vi "MAIN.vi"(6 "ECU TYPE":u16(ring) items=["LSMD", "LSMP", "LSMRL", "LSMRR"]) -> (0 "Data By ID OK":bool, 1 "Hall Test 3 OK":bool, 2 "Sleep Request OK":bool, 3 "Hall Test 1 OK":bool, 4 "SBC OK":bool, 5 "Hall Test 2 OK":bool, 7 "Hard Reset OK":bool, 8 "BIST OK":bool, 9 "SW Version OK":bool, 10 "ECU ID OK":bool, 11 "Session OK":bool)   [LabVIEW 2023]
uses:
  Sub VIs/Global .vi
panel:
  out "Numeric Request":i32=416962034 format="%x"
  out "ReplyTracMex":string
  out "Trazabilidad":bool
  in  "Trazabilidad\nOFF  /  ON":bool
  in  "Stop":bool
  in  "Start":bool
  out "Puerto DAQ":i32
  out "Respuesta Trazabilidad":string
  out "Finish Time":string
  out "Start Time":string
  out "Status":i8
  in  "Número Serial":string
  out "Enter Brose Ext OK":bool
  out "Hall Test 3 Response":string
  out "Enter Brose Ext":string
  out "ECU Hard Reset":string
  out "Program SBC":string
  out "ID Response":string
  out "ID Request":string
  out "Tester Present OK":bool
  out "Hall Test 2 Response":string
  out "Hall Test 1 Response":string
  out "Supply Voltage ADC Response":string
  out "Self Test BIST":string
  out "Sleep Request Response":string
  out "Read Data By ID":string
  out "Verify ECU ID String":string
  out "Verify SW Version":string
  out "Tester Present Command":string
  out "Enter Brose EOL Ext Session":string
  # "*Revisar debido a cambio en respuesta"
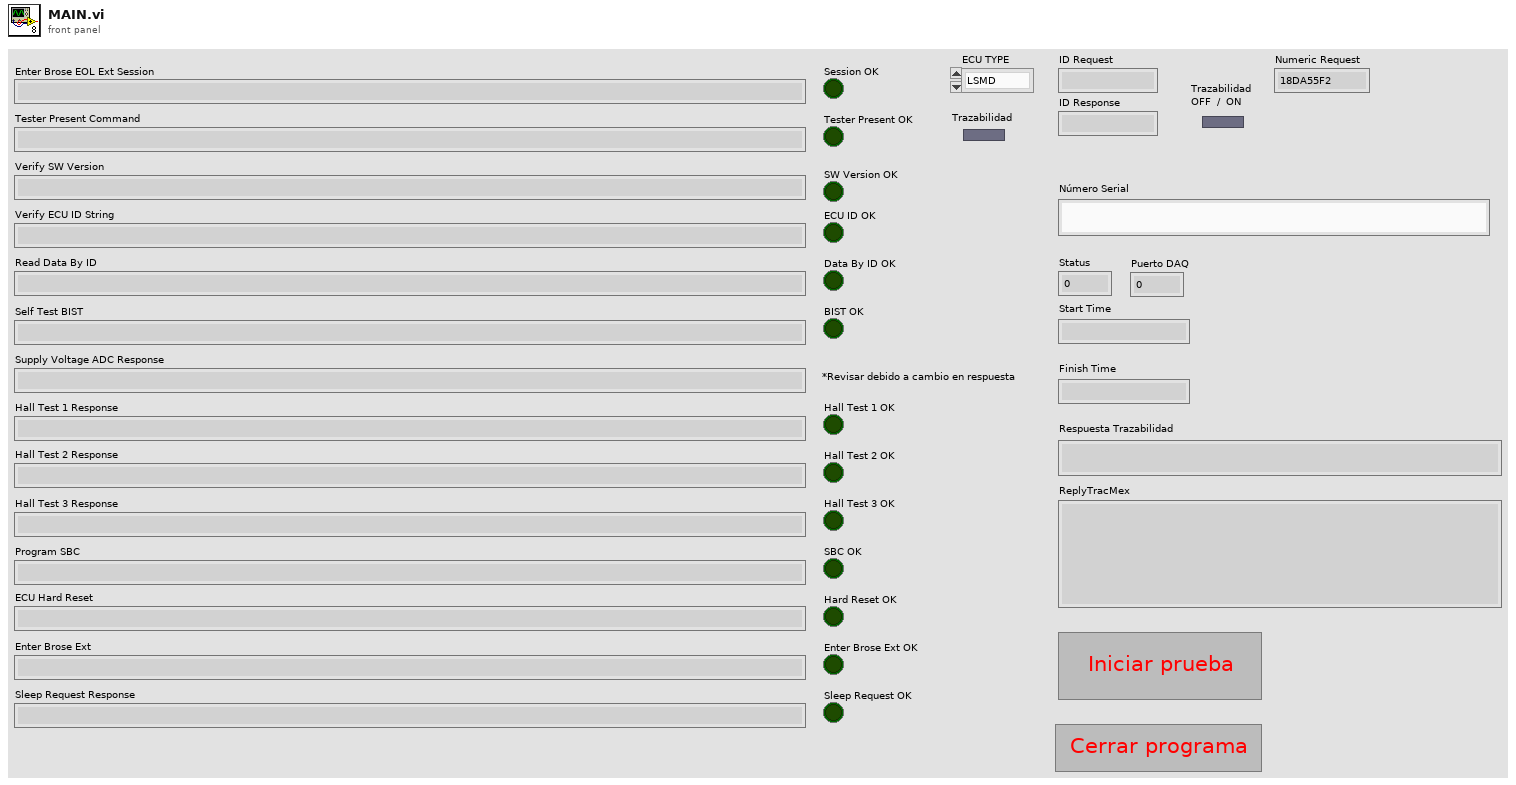
[diagram p1: front panel]
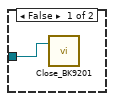
[diagram p2: hidden frame]
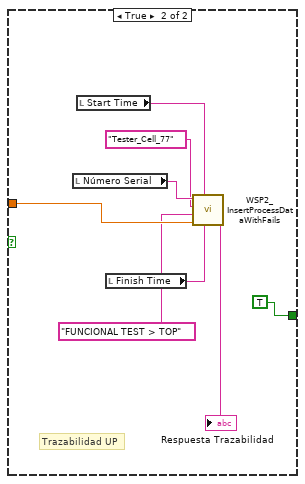
[diagram p3: hidden frame]
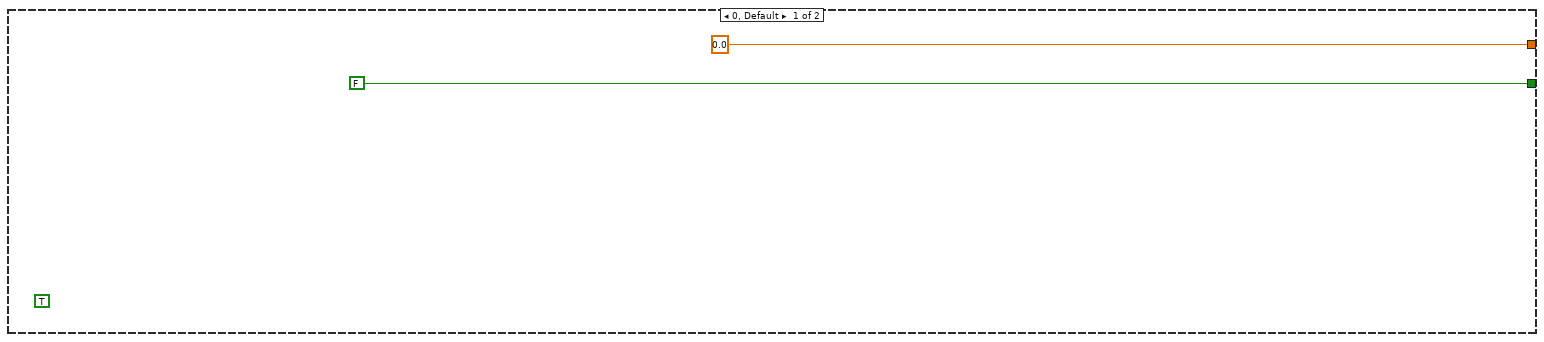
[diagram p4: hidden frame]
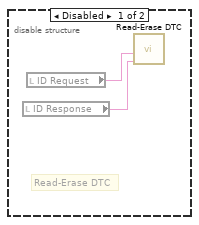
[diagram p7: hidden frame]
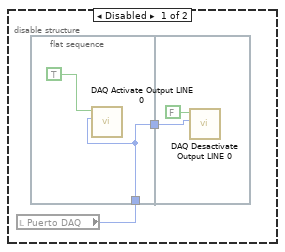
[diagram p8: hidden frame]
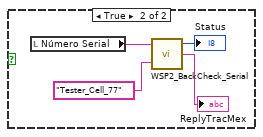
[diagram p9: hidden frame]
diagram:
  n1 = call "Initalization_BK9201.vi"("Instrument In"=refnum<visa-resource-name> "USB0::0x2EC7::0x9200::800889011776910056::INSTR") -> ("Instrument Out"=w1:refnum<visa-resource-name>)  [unwired: 3 in, 1 out]
  n2 = while {
    tunnel: w1 -> [w5]
    stop <- w4 stop-if-true
    n3 = while {
      tunnel: ["Stop"] -> w4
      tunnel: [w268] -> w3
      stop <- w273 stop-if-true
      n4 = Wait (ms)(milliseconds to wait=u32 100) -> ()  [unwired: 1 out]
      n5 = Select(t=FALSE, s="Stop", f=TRUE) -> (s? t:f=w268:bool)
      n6 = Or(x="Stop", y="Start") -> (x .or. y?=w273:bool)
      "Trazabilidad" <- "Trazabilidad\nOFF  /  ON"
    }
    n7 = case shown="True" w3 {
      tunnel: w5 -> [w6 w8]
      frame False {
        n8 = call "Close_BK9201.vi"("Instrument In"=w6) -> ()  [unwired: 2 in, 1 out]
      }
      frame True {
        n9 = flat-sequence {
          tunnel: w8 -> [w255]
          tunnel: [w257] -> w9
          tunnel: [w266] -> w7
          frame #0 {
            n10 = call "Display Message to User"("Message"="COLOCA LA PIEZA EN EL NIDO.\n\nCIERRA EL NIDO Y PRESIONA OK.") -> ()  [unwired: 9 in, 2 out]
          }
          frame #1 {
            w256 = u16 1 items=["Disable", "Enable"] ("Ring")
            n11 = call "Setting_BK9201.vi"("Instrument In"=w255, "Set Out Voltage"=9.0, "Current Limit"=1.0, "Ring"=w256) -> ("Instrument Out"=w257:refnum<visa-resource-name>)  [unwired: 14 in, 1 out]
          }
          frame #2 {
            n12 = local read "Trazabilidad"() -> (w260:bool)
            n13 = case shown="False" w260 {
              frame False {
                n14 = local write "Status"(i8 1 ("Status 2")) -> ()
              }
              frame True {
                n15 = local read "Número Serial"() -> (w264:string)
                n16 = call "WSP2_BackCheck_Serial.vi"("serialNumber"=w264, "stationName"="Tester_Cell_77") -> ("Status"=→"Status":i8, "ReplyTracMex"=→"ReplyTracMex":string)  [unwired: 1 out]
              }
            }
          }
          frame #3 {
            n17 = local read "Status"() -> (w266:i8)
          }
        }
        n18 = case shown="1" w7 {
          tunnel: [FALSE w25] -> w12
          tunnel: [0.0 ("f") w32] -> w11
          tunnel: w9 -> [_ w27]
          frame 0, Default {
            (unwired) TRUE
          }
          frame 1 {
            n19 = flat-sequence {
              tunnel: ["ECU TYPE"] -> w24
              tunnel: [w83] -> w68
              tunnel: [w82] -> w67
              tunnel: w24 -> [w77]
              tunnel: w68 -> [w92]
              tunnel: w67 -> [w91]
              tunnel: [w90] -> w66
              tunnel: [w89] -> w65
              tunnel: [w93] -> w64
              tunnel: [w94] -> w63
              tunnel: w66 -> [w96]
              tunnel: w65 -> [w95]
              tunnel: [w105] -> w62
              tunnel: [w106] -> w61
              tunnel: w64 -> [w108]
              tunnel: w63 -> [w107]
              tunnel: [w122] -> w59
              tunnel: [w121] -> w60
              tunnel: w62 -> [w124]
              tunnel: w61 -> [w123]
              tunnel: [w128] -> w58
              tunnel: [w127] -> w57
              tunnel: w60 -> [w129]
              tunnel: w59 -> [w130]
              tunnel: [w139] -> w29
              tunnel: [w138] -> w31
              tunnel: w58 -> [w134]
              tunnel: w57 -> [w133]
              tunnel: w31 -> [w146]
              tunnel: [w146] -> w30
              tunnel: w29 -> [w145]
              tunnel: [w145] -> w28
              tunnel: w27 -> [w141]
              tunnel: [w140] -> w26
              tunnel: w30 -> [w150]
              tunnel: w28 -> [w149]
              tunnel: [w148] -> w56
              tunnel: [w147] -> w55
              tunnel: [w160] -> w54
              tunnel: [w159] -> w53
              tunnel: w56 -> [w154]
              tunnel: w55 -> [w153]
              tunnel: w54 -> [w164]
              tunnel: w53 -> [w163]
              tunnel: [w162] -> w52
              tunnel: [w161] -> w51
              tunnel: [w174] -> w50
              tunnel: [w173] -> w49
              tunnel: w52 -> [w168]
              tunnel: w51 -> [w167]
              tunnel: w50 -> [w177]
              tunnel: w49 -> [w178]
              tunnel: [w176] -> w48
              tunnel: [w175] -> w47
              tunnel: [w188] -> w46
              tunnel: [w187] -> w45
              tunnel: w48 -> [w182]
              tunnel: w47 -> [w181]
              tunnel: [w190] -> w44
              tunnel: w46 -> [w190]
              tunnel: [w189] -> w43
              tunnel: w45 -> [w189]
              tunnel: [w198] -> w42
              tunnel: [w197] -> w41
              tunnel: w44 -> [w196]
              tunnel: w43 -> [w195]
              tunnel: w42 -> [w206]
              tunnel: w41 -> [w205]
              tunnel: [w204] -> w40
              tunnel: [w203] -> w39
              tunnel: w40 -> [w211]
              tunnel: [w211] -> w38
              tunnel: w39 -> [w210]
              tunnel: [w210] -> w37
              tunnel: w38 -> [w219]
              tunnel: w37 -> [w218]
              tunnel: [w215] -> w36
              tunnel: [w214] -> w35
              tunnel: [w225] -> w33
              tunnel: [w224] -> w34
              tunnel: w36 -> [w223]
              tunnel: w35 -> [w222]
              tunnel: w34 -> [w228]
              tunnel: w33 -> [w229]
              tunnel: w26 -> [w230]
              tunnel: [w243] -> w32
              tunnel: [w240] -> w25
              frame #0 {
                w70 = FALSE
                w69 = ""
                n20 = local write "Hard Reset OK"(w70) -> ()
                n21 = local write "Sleep Request OK"(w70) -> ()
                n22 = local write "Enter Brose Ext OK"(w70) -> ()
                n23 = local write "SBC OK"(w70) -> ()
                n24 = local write "ECU ID OK"(w70) -> ()
                n25 = local write "Data By ID OK"(w70) -> ()
                n26 = local write "SW Version OK"(w70) -> ()
                n27 = local write "Tester Present OK"(w70) -> ()
                n28 = local write "Session OK"(w70) -> ()
                n29 = local write "Hall Test 2 OK"(w70) -> ()
                n30 = local write "Hall Test 3 OK"(w70) -> ()
                n31 = local write "BIST OK"(w70) -> ()
                n32 = local write "Hall Test 1 OK"(w70) -> ()
                n33 = local write "Enter Brose EOL Ext Session"(w69) -> ()
                n34 = local write "Supply Voltage ADC Response"(w69) -> ()
                n35 = local write "Tester Present Command"(w69) -> ()
                n36 = local write "Sleep Request Response"(w69) -> ()
                n37 = local write "Enter Brose Ext"(w69) -> ()
                n38 = local write "Finish Time"(w69) -> ()
                n39 = local write "ECU Hard Reset"(w69) -> ()
                n40 = local write "Respuesta Trazabilidad"(w69) -> ()
                n41 = local write "Hall Test 1 Response"(w69) -> ()
                n42 = local write "ReplyTracMex"(w69) -> ()
                n43 = local write "Hall Test 3 Response"(w69) -> ()
                n44 = local write "Verify ECU ID String"(w69) -> ()
                n45 = local write "Program SBC"(w69) -> ()
                n46 = local write "Hall Test 2 Response"(w69) -> ()
                n47 = local write "Verify SW Version"(w69) -> ()
                n48 = local write "Start Time"(w69) -> ()
                n49 = local write "Read Data By ID"(w69) -> ()
                n50 = local write "Self Test BIST"(w69) -> ()
              }
              frame #1 {
                n51 = call "WSP2_GetDateTimeStr.vi"() -> ("Time"=→"Start Time":string)  [unwired: 1 in, 1 out]
              }
              frame #2 {
                # "ECU SELECT"
                n52 = global write "Global .vi" "ECU TYPE"("ECU TYPE") -> ()
                n53 = call "ECU Selector64.vi"("ECU TYPE"="ECU TYPE") -> ("ID Response"=→"ID Response":string, "Puerto DAQ"=→"Puerto DAQ":i32, "Numeric Request"=→"Numeric Request":i32, "ID Request"=→"ID Request":string)  [unwired: 1 in, 1 out]
              }
              frame #3 {
                # "Comunication Startup"
                n54 = local read "ID Request"() -> (w80:string)
                n55 = local read "ID Response"() -> (w79:string)
                n56 = call "Session Request - Brose Session.vi"("ID Request"=w80, "ECU TYPE"=w77, "ID Response"=w79) -> ("Data String"=w81:string, "Write"=w83:refnum<k21>, "Read"=w82:refnum<k21>)  [unwired: 1 out]
                "Enter Brose EOL Ext Session" <- w81
                n57 = call "Evaluate Session.vi"("String In"=w81) -> ("Test OK"=→"Session OK":bool)
              }
              frame #4 {
                # "Tester Present Command"
                n58 = local read "ID Response"() -> (w85:string)
                n59 = local read "Numeric Request"() -> (w84:i32)
                n60 = local read "ID Request"() -> (w86:string)
                n61 = call "Tester Present Command.vi"("Numeric Request"=w84, "ID Response"=w85, "ID Request"=w86, "Read"=w91, "Write"=w92) -> ("Read out"=w90:refnum<k21>, "Write out"=w89:refnum<k21>, "Data String 2"=w88:string)  [unwired: 1 out]
                "Tester Present Command" <- w88
                n62 = call "Evaluate Tester Present.vi"("String In"=w88) -> ("Test OK"=→"Tester Present OK":bool)
              }
              frame #5 {
                n63 = disable-structure shown="Disabled" {
                  disable-tunnel: w96 -> [w104 _]
                  disable-tunnel: w95 -> [w103 _]
                  disable-tunnel: [w102 _] -> w94
                  disable-tunnel: [w101 _] -> w93
                  frame Disabled {
                    # "Verify SW Version"
                    n64 = local read "ID Response"() -> (w97:string)
                    n65 = local read "ID Request"() -> (w98:string)
                    n66 = call "Verify SW Version.vi"("ID Response"=w97, "ID Request"=w98, "Read"=w104, "Write"=w103) -> ("Data String 3"=w100:string, "Write out"=w102:refnum<k21>, "Read out"=w101:refnum<k21>)  [unwired: 1 out]
                    "Verify SW Version" <- w100
                    n67 = call "Evaluate SW Version Response.vi"("String In"=w100) -> ("Test OK"=→"SW Version OK":bool)
                  }
                  frame Enabled {
                  }
                }
              }
              frame #6 {
                n68 = disable-structure shown="Disabled" {
                  disable-tunnel: w108 -> [w116 _]
                  disable-tunnel: w107 -> [w115 _]
                  disable-tunnel: [w114 _] -> w106
                  disable-tunnel: [w113 _] -> w105
                  frame Disabled {
                    # "Verify ECU ID String"
                    n69 = local read "ID Response"() -> (w111:string)
                    n70 = local read "ID Request"() -> (w112:string)
                    n71 = call "Verify ECU ID String.vi"("ID Response"=w111, "ID Request"=w112, "Read"=w116, "Write"=w115) -> ("Data String 3"=w110:string, "Write out"=w114:refnum<k21>, "Read out"=w113:refnum<k21>)  [unwired: 1 out]
                    "Verify ECU ID String" <- w110
                    n72 = call "Evaluate ECU ID String.vi"("String In"=w110) -> ("Test OK"=→"ECU ID OK":bool)
                  }
                  frame Enabled {
                  }
                }
              }
              frame #7 {
                # "Start Routine Read Data By ID"
                n73 = local read "ID Response"() -> (w119:string)
                n74 = local read "ID Request"() -> (w120:string)
                n75 = call "Start Routine - Read Data ID.vi"("ID Response"=w119, "ID Request"=w120, "Read"=w124, "Write"=w123) -> ("Data String 3"=w118:string, "Write out"=w122:refnum<k21>, "Read out"=w121:refnum<k21>)  [unwired: 1 out]
                "Read Data By ID" <- w118
                n76 = call "Evaluate Read Data By ID.vi"("String In"=w118) -> ("Test OK"=→"Data By ID OK":bool)
              }
              frame #8 {
                # "Selt Test BIST"
                n77 = local read "ID Response"() -> (w131:string)
                n78 = local read "ID Request"() -> (w132:string)
                n79 = call "Self Test BIST.vi"("ID Response"=w131, "ID Request"=w132, "Read"=w129, "Write"=w130) -> ("Data String 3"=w125:string, "Write out"=w127:refnum<k21>, "Read out"=w128:refnum<k21>)  [unwired: 1 out]
                "Self Test BIST" <- w125
                n80 = call "Evaluate Self Test BIST.vi"("String In"=w125) -> ("Test OK"=→"BIST OK":bool)
              }
              frame #9 {
                # "Supply Voltage ADC Measurement"
                n81 = local read "ID Response"() -> (w135:string)
                n82 = local read "ID Request"() -> (w136:string)
                n83 = call "Supply Voltage ADC Measurement.vi"("ID Response"=w135, "ID Request"=w136, "Read"=w134, "Write"=w133) -> ("Data String 3"=→"Supply Voltage ADC Response":string, "Write out"=w139:refnum<k21>, "Read out"=w138:refnum<k21>)  [unwired: 1 out]
              }
              frame #10 {
                w142 = u16 1 items=["Disable", "Enable"] ("Ring")
                n84 = call "Setting_BK9201.vi"("Instrument In"=w141, "Set Out Voltage"=12.0, "Current Limit"=1.0, "Ring"=w142) -> ("Instrument Out"=w140:refnum<visa-resource-name>)  [unwired: 14 in, 1 out]
              }
              frame #11 {
                # "Display Message I"
                n85 = global read "Global .vi" "ECU TYPE"() -> (w152:u16)
                n86 = call "Cuadro de Texto.vi"("Numeric"=1.0, "Read"=w150, "Write"=w149, "ECU TYPE"=w152) -> ("Write out"=w147:refnum<k21>, "Read out"=w148:refnum<k21>)
              }
              frame #12 {
                # "Hall Test 1"
                n87 = local read "ID Response"() -> (w157:string)
                n88 = local read "ID Request"() -> (w158:string)
                n89 = call "Hall Test.vi"("ID Response"=w157, "ID Request"=w158, "Read"=w154, "Write"=w153) -> ("Data String 3"=w156:string, "Write out"=w159:refnum<k21>, "Read out"=w160:refnum<k21>)  [unwired: 1 out]
                "Hall Test 1 Response" <- w156
                n90 = call "Evaluate Hall Test 1.vi"("String In"=w156) -> ("Test OK"=→"Hall Test 1 OK":bool)
              }
              frame #13 {
                # "Display Message II"
                n91 = global read "Global .vi" "ECU TYPE"() -> (w166:u16)
                n92 = call "Cuadro de Texto.vi"("Numeric"=2.0, "Read"=w164, "Write"=w163, "ECU TYPE"=w166) -> ("Write out"=w161:refnum<k21>, "Read out"=w162:refnum<k21>)
              }
              frame #14 {
                # "Hall Test 2"
                n93 = local read "ID Response"() -> (w171:string)
                n94 = local read "ID Request"() -> (w172:string)
                n95 = call "Hall Test.vi"("ID Response"=w171, "ID Request"=w172, "Read"=w168, "Write"=w167) -> ("Data String 3"=w170:string, "Write out"=w174:refnum<k21>, "Read out"=w173:refnum<k21>)  [unwired: 1 out]
                "Hall Test 2 Response" <- w170
                n96 = call "Evaluate Hall Test 2.vi"("String In"=w170) -> ("Test OK"=→"Hall Test 2 OK":bool)
              }
              frame #15 {
                # "Display Mesagge III"
                n97 = global read "Global .vi" "ECU TYPE"() -> (w180:u16)
                n98 = call "Cuadro de Texto.vi"("Numeric"=3.0, "Read"=w178, "Write"=w177, "ECU TYPE"=w180) -> ("Write out"=w175:refnum<k21>, "Read out"=w176:refnum<k21>)
              }
              frame #16 {
                # "Hall Test 3"
                n99 = local read "ID Request"() -> (w186:string)
                n100 = local read "ID Response"() -> (w185:string)
                n101 = call "Hall Test.vi"("ID Response"=w185, "ID Request"=w186, "Read"=w182, "Write"=w181) -> ("Data String 3"=w184:string, "Write out"=w187:refnum<k21>, "Read out"=w188:refnum<k21>)  [unwired: 1 out]
                "Hall Test 3 Response" <- w184
                n102 = call "Evaluate Hall Test 3.vi"("String In"=w184) -> ("Test OK"=→"Hall Test 3 OK":bool)
              }
              frame #17 {
                n103 = disable-structure shown="Enabled" {
                  frame Disabled {
                    # "Read-Erase DTC"
                    n104 = local read "ID Response"() -> (w191:string)
                    n105 = local read "ID Request"() -> (w192:string)
                    n106 = call "Read-Erase DTC.vi"("ID Response"=w191, "ID Request"=w192) -> ()  [unwired: 2 in, 4 out]
                  }
                  frame Enabled {
                  }
                }
              }
              frame #18 {
                # "Program SBC"
                n107 = local read "ID Response"() -> (w199:string)
                n108 = local read "ID Request"() -> (w200:string)
                n109 = call "Routine Before BIST.vi"("ID Response"=w199, "ID Request"=w200, "Read"=w196, "Write"=w195) -> ("Data String 3"=w194:string, "Write out"=w197:refnum<k21>, "Read out"=w198:refnum<k21>)  [unwired: 1 out]
                "Program SBC" <- w194
                n110 = call "Evaluate SBC.vi"("String In"=w194) -> ("Test OK"=→"SBC OK":bool)
              }
              frame #19 {
                # "ECU Hard Reset"
                n111 = local read "ID Request"() -> (w207:string)
                n112 = local read "ID Response"() -> (w208:string)
                n113 = call "Routine Before BIST I.vi"("ID Response"=w208, "ID Request"=w207, "Read"=w206, "Write"=w205) -> ("Data String 3"=w202:string, "Write out"=w204:refnum<k21>, "Read out"=w203:refnum<k21>)  [unwired: 1 out]
                "ECU Hard Reset" <- w202
                n114 = call "Evaluate ECU Hard Reset.vi"("String In"=w202) -> ("Test OK"=→"Hard Reset OK":bool)
              }
              frame #20 {
                n115 = Wait (ms)(milliseconds to wait=u32 500) -> ()  [unwired: 1 out]
              }
              frame #21 {
                n116 = local read "ID Request"() -> (w217:string)
                n117 = local read "ID Response"() -> (w216:string)
                n118 = call "Session Request II.vi"("ID Response"=w216, "ID Request"=w217, "Read"=w218, "Write"=w219) -> ("Data String 3"=w213:string, "Write out"=w215:refnum<k21>, "Read out"=w214:refnum<k21>)  [unwired: 1 out]
                "Enter Brose Ext" <- w213
                n119 = call "Evaluate Session.vi"("String In"=w213) -> ("Test OK"=→"Enter Brose Ext OK":bool)
              }
              frame #22 {
                # "Sleep Current Measurement"
                n120 = local read "ID Request"() -> (w227:string)
                n121 = local read "ID Response"() -> (w226:string)
                n122 = call "Sleep Request.vi"("ID Response"=w226, "ID Resquest"=w227, "Read"=w222, "Write"=w223) -> ("Data String 3"=w221:string, "Write out"=w224:refnum<k21>, "Read out"=w225:refnum<k21>)  [unwired: 1 out]
                "Sleep Request Response" <- w221
                n123 = call "Evaluate Sleep Request.vi"("String In"=w221) -> ("Test OK"=→"Sleep Request OK":bool)
              }
              frame #23 {
                # "Cierra y\nlimpia puerto\nCAN"
                n124 = call <vilib>:"XNET Clear.vi"("session in"=w229) -> ()  [unwired: 14 in, 1 out]
                n125 = call <vilib>:"XNET Clear.vi"("session in"=w228) -> ()  [unwired: 14 in, 1 out]
              }
              frame #24 {
                w232 = u16 0 items=["Disable", "Enable"] ("Ring")
                # "Desactiva fuente"
                n126 = call "Setting_BK9201.vi"("Instrument In"=w230, "Set Out Voltage"=0.0, "Ring"=w232) -> ()  [unwired: 15 in, 2 out]
              }
              frame #25 {
                # "Descarga de capacitor"
                n127 = disable-structure shown="Enabled" {
                  frame Disabled {
                    n128 = local read "Puerto DAQ"() -> (w233:i32)
                    n129 = flat-sequence {
                      tunnel: w233 -> [w235]
                      tunnel: [w235] -> w234
                      tunnel: w234 -> [w237]
                      frame #0 {
                        n130 = call "DAQ Activate Output LINE 0.vi"("Puerto"=w235, "data"=TRUE) -> ()  [unwired: 4 in, 2 out]
                      }
                      frame #1 {
                        n131 = call "DAQ Desactivate Output LINE 0.vi"("Puerto"=w237, "data"=FALSE) -> ()  [unwired: 4 in, 2 out]
                      }
                    }
                  }
                  frame Enabled {
                  }
                }
              }
              frame #26 {
                # "Recibe tiempo final de prueba"
                n132 = call "WSP2_GetDateTimeStr.vi"() -> ("Time"=→"Finish Time":string)  [unwired: 1 in, 1 out]
              }
              frame #27 {
                # "Revivisa que haya pasado las pruebas"
                n133 = local read "Data By ID OK"() -> (w248:bool)
                n134 = local read "ECU ID OK"() -> (w249:bool)
                n135 = local read "Sleep Request OK"() -> (w241:bool)
                n136 = local read "SW Version OK"() -> (w250:bool)
                n137 = local read "BIST OK"() -> (w247:bool)
                n138 = local read "Session OK"() -> (w251:bool)
                n139 = local read "SBC OK"() -> (w242:bool)
                n140 = Compound Arithmetic op=AND(w251, w250, w249, w248, w247, w242, w241) -> (w246:bool)
                n141 = Select(t=1.0, s=w246, f=0.0) -> (s? t:f=w243:dbl)
                n142 = local read "Trazabilidad"() -> (w240:bool)
              }
            }
          }
        }
        n143 = case shown="False" w12 {
          tunnel: w11 -> [_ w17]
          tunnel: [TRUE TRUE] -> w10
          frame False {
            # "Trazabilidad UP"
          }
          frame True {
            # "Trazabilidad UP"
            n144 = local read "Número Serial"() -> (w21:string)
            n145 = local read "Start Time"() -> (w19:string)
            n146 = local read "Finish Time"() -> (w18:string)
            n147 = call "WSP2_InsertProcessDataWithFails.vi"("EndTime"=w18, "EntryTime"=w19, "PassFail"=w17, "ProcessName"="FUNCIONAL TEST > TOP", "StationName"="Tester_Cell_77", "SerialNumber"=w21) -> ("ReplyTrace"=→"Respuesta Trazabilidad":string)  [unwired: 4 in, 1 out]
          }
        }
        n148 = flat-sequence {
          tunnel: w10 -> [w252]
          frame #0 {
            # "Mensaje de retirar pieza"
            n149 = call "Display Message to User2"("Enable"=w252, "Message"="RETIRE LA PIEZA DEL NIDO") -> ()  [unwired: 8 in, 2 out]
          }
        }
      }
    }
  }
